vi "Gyro steer.vi"(8 "Turn Speed":dbl, 9 "Target Angle":dbl, 11 "Changed?":bool) -> (1 "In Range?":bool, 3 "X out":dbl)   [LabVIEW 2015]
uses:
  Robot Global Data.vi
  <vilib>/addons/control/pid/pid.llb/PID (DBL).vi
  <vilib>/addons/control/pid/NI_PID_pid.lvlib
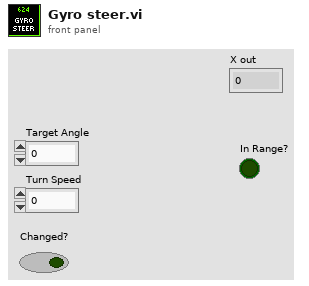
[diagram p1: front panel]
types:
  T1 = typedef "Dashboard Control Data.ctl" = cluster{"Auton Loops":dbl, "Shooter Presets":T2, "Encoder Control":T4, "Steer PID output":cluster{"output high":dbl, "output low":dbl}, " Steer PID gains":cluster{"proportional gain (Kc)":dbl, "integral time (Ti, min)":dbl, "derivative time (Td, min)":dbl}, "Drivetrain Settings":T5}
  T2 = typedef "Shooter Presets.ctl" = cluster{"Batter Shot":T3, "Low Bar Curve Shot":T3, "Deep Middle Shot":T3, "Manual Shot":T3}
  T3 = typedef "Shot Presets.ctl" = cluster{"Left Wheel RPM":dbl, "Right Wheel RPM":dbl}
  T4 = typedef "Encoder Control.ctl" = cluster{"Right Tick Constat":dbl, "Left Tick Constant":dbl, "Reset?":bool, "Y Dist":cluster{"PID gains":cluster{"proportional gain (Kc)":dbl, "integral time (Ti, min)":dbl, "derivative time (Td, min)":dbl}}, "Y Stop Thresh":dbl, "Y Stop Speed":dbl}
  T5 = typedef "Drivetrain Settings.ctl" = cluster{"Gyro Tolerance":dbl, "Throttle Ramp (ms)":dbl, "Angular rate compensation":bool, "Throttle to Rate Scale":dbl, "Rate compensation gain":dbl}
  T6 = cluster{"proportional gain (Kc)":dbl, "integral time (Ti, min)":dbl, "derivative time (Td, min)":dbl}
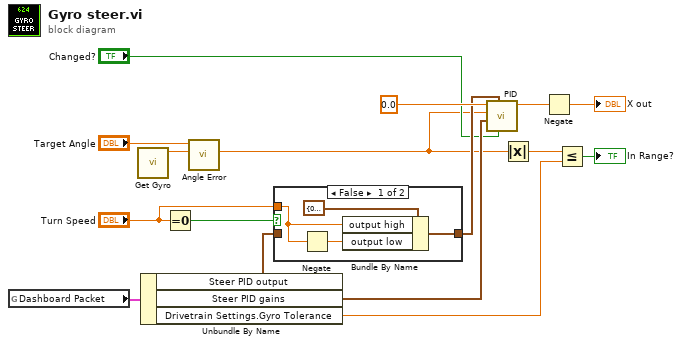
[diagram p0: block diagram]
diagram:
  n1 = global read "Robot Global Data.vi" "Dashboard Packet"() -> (w16:T1)
  n2 = call "Get Gyro.vi"() -> ("Angle"=w6:dbl)  [unwired: 11 in]
  n3 = Unbundle By Name(w16) -> ("Steer PID output"=w13:cluster{"output high":dbl, "output low":dbl}, "Steer PID gains"=w10:T6, "Drivetrain Settings.Gyro Tolerance"=w2:dbl)
  n4 = Equal To 0?(x="Turn Speed") -> (x = 0?=w15:bool)
  n5 = call "Angle Error.vi"("Angle"=w6, "Target Angle"="Target Angle") -> ("Error"=w4:dbl)  [unwired: 9 in]
  n6 = case shown="False" w15 {
    tunnel: "Turn Speed" -> [w18 _]
    tunnel: w13 -> [_ w21]
    tunnel: [w20 w21] -> w9
    frame False {
      n7 = Negate(x=w18) -> (-x=w19:dbl)
      n8 = Bundle By Name(cluster=cluster{"output high":dbl, "output low":dbl} {"output high"=0.0, "output low"=0.0} ("Steer PID output Range"), "output high"=w18, "output low"=w19) -> (w20:cluster{"output high":dbl, "output low":dbl})
    }
    frame True {
    }
  }
  n9 = call-poly <vilib>:"PID.vi"("reinitialize? (F)"="Changed?", "output range"=w9, "PID gains"=w10, "process variable"=w4, "setpoint"=0.0) -> ("output"=w7:dbl)  [unwired: 5 in, 1 out]
  n10 = Absolute Value(x=w4) -> (abs(x)=w3:dbl)
  n11 = Negate(x=w7) -> (-x=→"X out":dbl)
  n12 = Less Or Equal?(x=w3, y=w2) -> (x <= y?=→"In Range?":bool)
